vi "Pulse Simulation.vi"() -> ()   [LabVIEW 2011]
panel:
  in  "Start 2":bool
  in  "Time 2":u32(slide)=500 scale=0.0..2000.0
  out "Elapsed 2":u32
  out "Timeout 2":bool
  out "Elapsed":u32
  out "Timeout":bool
  in  "Time":u32(slide)=500 scale=0.0..2000.0
  in  "Start":bool
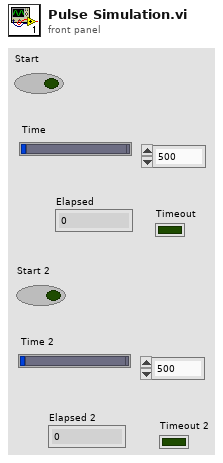
[diagram p1: front panel]
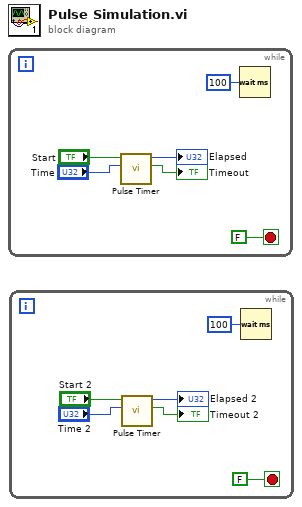
[diagram p0: block diagram]
diagram:
  n1 = while {
    stop <- FALSE stop-if-true
    n2 = call "Pulse Timer.vi"("Time"="Time", "Start"="Start") -> ("Timeout"=→"Timeout":bool, "Elapsed"=→"Elapsed":u32)  [unwired: 8 in]
    n3 = Wait (ms)(milliseconds to wait=u32 100) -> ()  [unwired: 1 out]
  }
  n4 = while {
    stop <- FALSE stop-if-true
    n5 = call "Pulse Timer.vi"("Time"="Time 2", "Start"="Start 2") -> ("Timeout"=→"Timeout 2":bool, "Elapsed"=→"Elapsed 2":u32)  [unwired: 8 in]
    n6 = Wait (ms)(milliseconds to wait=u32 100) -> ()  [unwired: 1 out]
  }
